vi "Pre Launch Init.vi"(11 "Cli in":refnum<class "Cli.lvclass">) -> (0 "error out":errorcluster, 3 "Cli out":refnum<class "Cli.lvclass">)   [LabVIEW 2022 SP3, in "Cli.lvlib" / "Cli.lvclass"]
doc: "(<B>Filename</B>: Actor Framework.lvlib:Actor.lvclass:Pre Launch Init.vi)\n\nDefines behavior that occurs after the Launch Actor method is invoked but before the actor's Actor Core method begins running.\n\nThe Pre Launch Init method is guaranteed to finish before the Launch Actor method returns to its caller and before the actor itself receives any messages. Any references that the Pre Launch Init method obtains are guaranteed to have the same lifetime as the actor itself. Any errors that the Pre Launch Init method returns will abort the launch.\n\nBy default, this method does nothing. A descendant class may override it to define behavior."
uses:
  Cli.lvclass
  Cli.lvclass/Cli.ctl
  <vilib>/ActorFramework/Actor/Actor.lvclass
  ArgumentParser/Source/ArgumentParser/ArgumentParser.lvclass
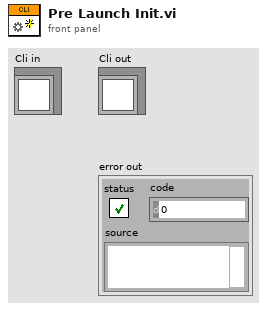
[diagram p1: front panel]
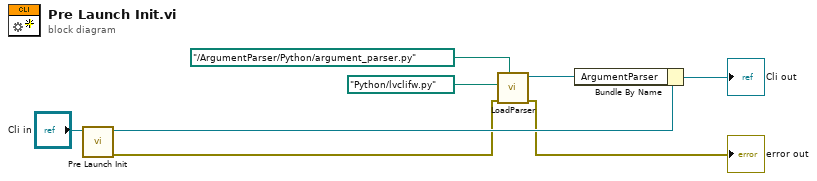
[diagram p0: block diagram]
diagram:
  n1 = call-parent "Pre Launch Init.vi"("Actor in"="Cli in") -> ("error out"=w3:errorcluster, "Actor out"=w7:refnum<class "Cli.lvclass">)  [unwired: 9 in]
  n2 = call "LoadParser.vi"("ModulePath"=path "../ArgumentParser/Python/argument_parser.py", "error in (no error)"=w3, "ParserPath"=path "Python/lvclifw.py") -> ("error out"=→"error out":errorcluster, "ArgumentParser"=w4:refnum<class "ArgumentParser.lvclass">)  [unwired: 7 in]
  n3 = Bundle By Name(cluster=w7, "ArgumentParser"=w4) -> (→"Cli out":refnum<class "Cli.lvclass">)
